vi "rs3 init all2.vi"(8 "error in":errorcluster, 10 "Select Device":i32, 11 "Select Sensor":i32) -> (0 "error out":errorcluster, 1 "Adv. enable?":i32, 2 "init results":T3, 3 "init error":string, 4 "All Devices":T2(array[cluster]), 5 "Sensor Array":T1(array[cluster]), 7 "Found RealSense":bool)   [LabVIEW 2019, in "libRealSense3.lvlib"]
doc: "Initialized the RealSense device. \nSelect the specific DEVICE and its specific SENSOR. \n\n\nINPUT:\nSelect Device The INDEX to the specific DEVICE handle\nSelect Sensor The INDEX to the specific SENSOR that is part of the selected DEVICE.\n \nOUTPUT:\ninit result Contains all the information about the selected device and its sensor. You will need to use the Dev Out HANDLE to communicate with the device. \n \nselected sensor array Contains the arrays of SENSORS attached to a specific DEVICE.\nall devices Contains array of all device that are attached to the PC."
uses:
  libRealSense3.lvlib
panel:
  # "RS3 Init All"
  # "(C) Intel Corp. 2017,  AGJ"
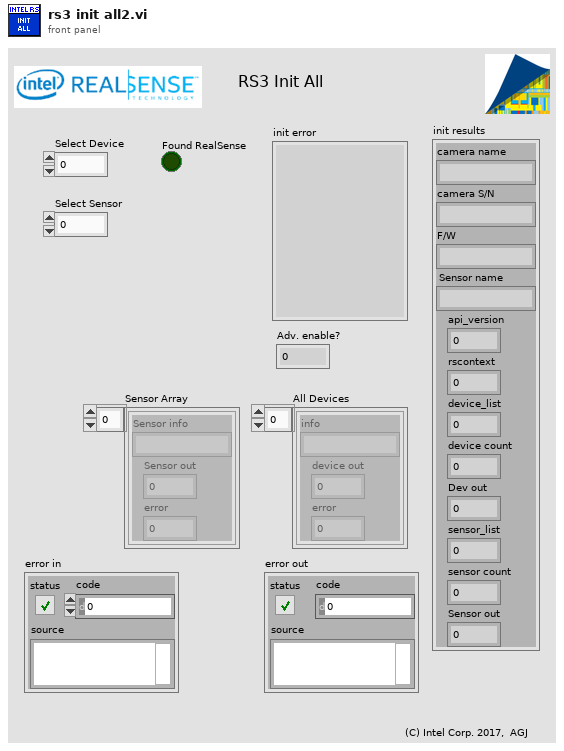
[diagram p1: front panel]
types:
  T1 = cluster{"Sensor info":string, "Sensor out":u64, "error":u64}[]
  T2 = cluster{"info":string, "device out":u64, "error":u64}[]
  T3 = cluster{"camera name":string, "camera S/N":string, "F/W":string, "Sensor name":string, "api_version":i32, "rscontext":u64, "device_list":u64, "device count":i32, "Dev out":u64, "sensor_list":u64, "sensor count":i32, "Sensor out":u64}
  T4 = cluster{"info":string, "device out":u64, "error":u64}
  T5 = cluster{"info":string, "info":string, "info":string, "Sensor info":string, "api_version":i32, "rscontext":u64, "device_list":u64, "device count":i32, "device out":u64, "sensor_list":u64, "sensor count":i32, "Sensor out":u64}
  T6 = cluster{"Sensor info":string, "Sensor out":u64, "error":u64}
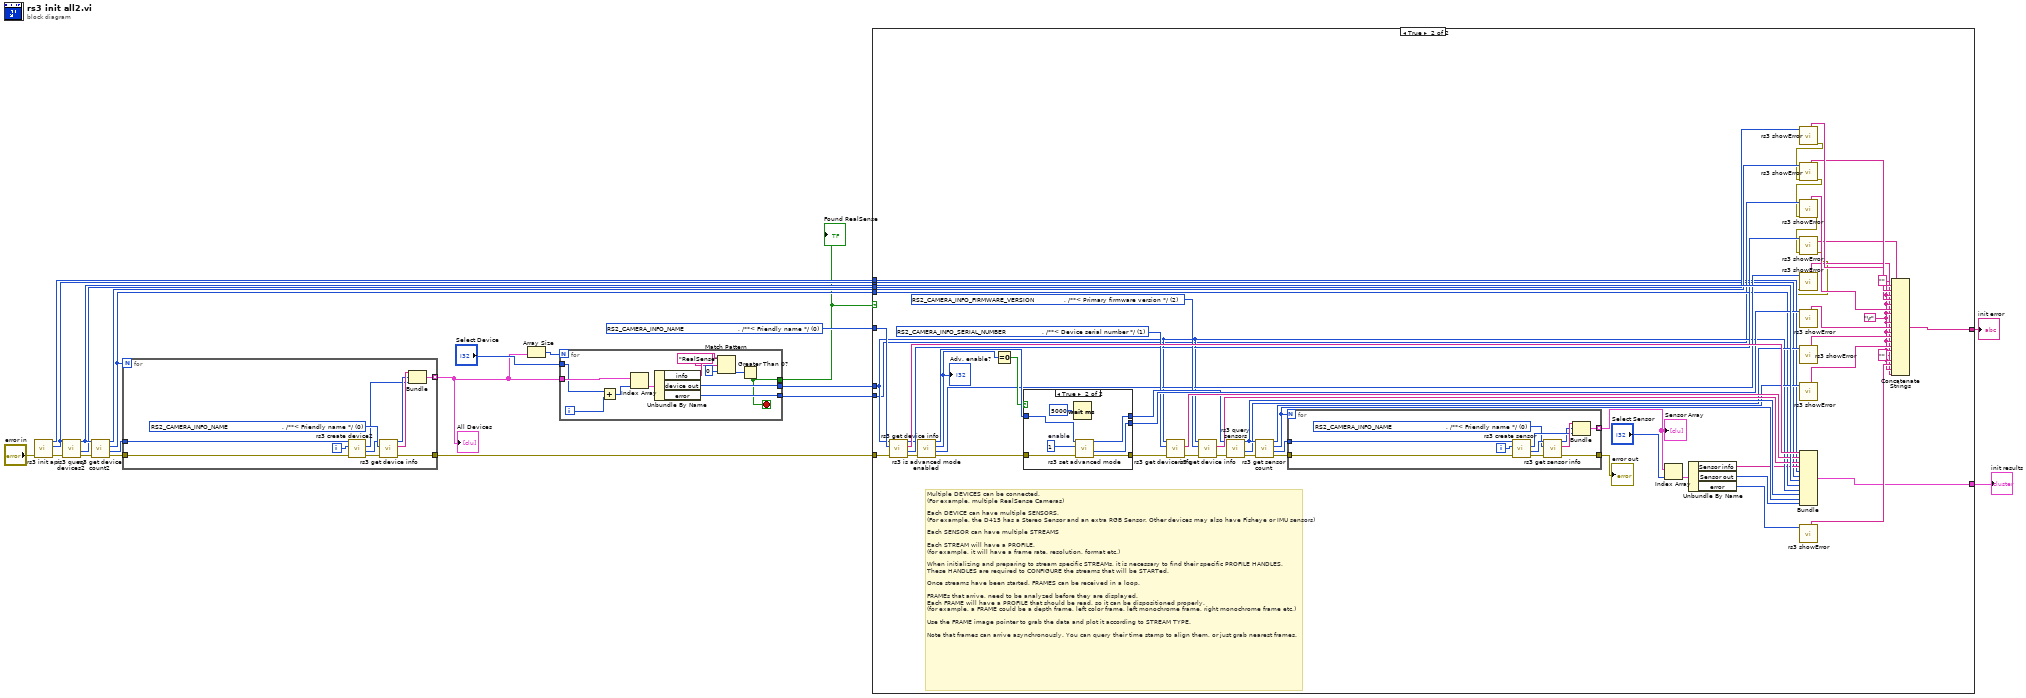
[diagram p0: block diagram]
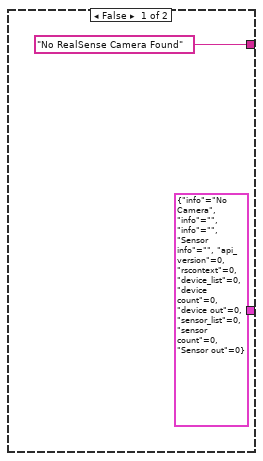
[diagram p2: hidden frame]
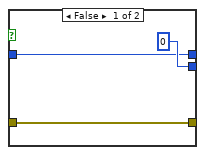
[diagram p3: hidden frame]
diagram:
  w20 = u16 0 items=["    RS2_CAMERA_INFO_NAME                           , /**< Friendly name */", "    RS2_CAMERA_INFO_SERIAL_NUMBER                  , /**< Device serial number */", "    RS2_CAMERA_INFO_FIRMWARE_VERSION               , /**< Primary firmware version */", "    RS2_CAMERA_INFO_PHYSICAL_PORT                       , /**< Unique identifier of the port the device is connected to (platform specific) */", "    RS2_CAMERA_INFO_DEBUG_OP_CODE                  , /**< If device supports firmware logging, this is the command to send to get logs from firmware */", "    RS2_CAMERA_INFO_ADVANCED_MODE                  , /**< True iff the device is in advanced mode */", "    RS2_CAMERA_INFO_PRODUCT_ID                     , /**< Product ID as reported in the USB descriptor */", "    RS2_CAMERA_INFO_CAMERA_LOCKED                  , /**< True iff EEPROM is locked */", "    RS2_CAMERA_INFO_COUNT                            /**< Number of enumeration values. Not a valid input: intended to be used in for-loops. */"] ("RS Camera info")
  n1 = call "rs3 init api.vi"("error in (no error)"="error in") -> ("error out"=w9:errorcluster, "rscontext"=w7:u64, "api_version"=w6:i32)  [unwired: 7 in, 1 out]
  n2 = call "rs3 query devices2.vi"("error in (no error)"=w9, "rscontext"=w7) -> ("error out"=w18:errorcluster, "error"=w17:u64, "device_list"=w21:u64)  [unwired: 7 in]
  n3 = call "rs3 get device count2.vi"("error in"=w18, "device_list"=w21) -> ("error out"=w12:errorcluster, "device_list_out"=w15:u64, "device count"=w16:i32, "error"=w19:u64)  [unwired: 6 in]
  n4 = for {
    N: w16 -> [_]
    tunnel: w15 -> [w32]
    tunnel: [w26] -> w1 mode=indexing
    tunnel: w12 -> [w25]
    tunnel: [w24] -> w11
    i -> [w31]
    w29 = u16 0 items=["    RS2_CAMERA_INFO_NAME                           , /**< Friendly name */", "    RS2_CAMERA_INFO_SERIAL_NUMBER                  , /**< Device serial number */", "    RS2_CAMERA_INFO_FIRMWARE_VERSION               , /**< Primary firmware version */", "    RS2_CAMERA_INFO_PHYSICAL_PORT                       , /**< Unique identifier of the port the device is connected to (platform specific) */", "    RS2_CAMERA_INFO_DEBUG_OP_CODE                  , /**< If device supports firmware logging, this is the command to send to get logs from firmware */", "    RS2_CAMERA_INFO_ADVANCED_MODE                  , /**< True iff the device is in advanced mode */", "    RS2_CAMERA_INFO_PRODUCT_ID                     , /**< Product ID as reported in the USB descriptor */", "    RS2_CAMERA_INFO_CAMERA_LOCKED                  , /**< True iff EEPROM is locked */", "    RS2_CAMERA_INFO_COUNT                            /**< Number of enumeration values. Not a valid input: intended to be used in for-loops. */"] ("RS Camera info")
    n5 = call "rs3 create device2.vi"("error in (no error)"=w25, "Device index"=w31, "device list in"=w32) -> ("error out"=w30:errorcluster, "Dev out"=w23:u64, "error"=w22:u64)  [unwired: 5 in, 1 out]
    n6 = call "rs3 get device info.vi"("error in (no error)"=w30, "RS Camera info"=w29, "device in"=w23) -> ("error out"=w24:errorcluster, "info"=w28:string, "device out"=w27:u64)  [unwired: 5 in, 1 out]
    n7 = Bundle("info"=w28, "device out"=w27, "error"=w22) -> (w26:T4)  [unwired: 1 in]
  }
  "All Devices" <- w1
  n8 = Array Size(array=w1) -> (size(s)=w2:i32)
  n9 = for {
    N: w2 -> [_]
    tunnel: w1 -> [w44]
    tunnel: "Select Device" -> [w35]
    tunnel: [w42] -> w13
    tunnel: [w41] -> w10
    tunnel: [w33] -> w5
    i -> [w36]
    stop <- w33 stop-if-true
    n10 = Add(x=w35, y=w36) -> (x+y=w37:i32)
    n11 = Index Array(array=w44, index=w37) -> (element=w43:T4)
    n12 = Unbundle By Name(w43) -> ("info"=w39:string, "device out"=w42:u64, "error"=w41:u64)
    n13 = Match Pattern(string=w39, regular expression="RealSense" ("string"), offset (0)=0) -> (offset past match=w34:i32)  [unwired: 3 out]
    n14 = Greater Than 0?(x=w34) -> (x > 0?=w33:bool)
  }
  "Found RealSense" <- w5
  n15 = case shown="True" w5 {
    tunnel: w21 -> [_ w104]
    tunnel: w20 -> [_ w91]
    tunnel: w19 -> [_ w89]
    tunnel: w17 -> [_ w88]
    tunnel: w16 -> [_ w70]
    tunnel: w13 -> [_ w69]
    tunnel: w11 -> [_ w68]
    tunnel: w10 -> [_ w67]
    tunnel: w7 -> [_ w56]
    tunnel: w6 -> [_ w55]
    tunnel: ["No RealSense Camera Found" w54] -> w4
    tunnel: [T5 {"info"="No Camera", "info"="", "info"="", "Sensor info"="", "api_version"=0, "rscontext"=0, "device_list"=0, "device count"=0, "device out"=0, "sensor_list"=0, "sensor count"=0, "Sensor out"=0} w53] -> w3
    frame False {
    }
    frame True {
      w72 = "\r"
      w98 = u16 2 items=["    RS2_CAMERA_INFO_NAME                           , /**< Friendly name */", "    RS2_CAMERA_INFO_SERIAL_NUMBER                  , /**< Device serial number */", "    RS2_CAMERA_INFO_FIRMWARE_VERSION               , /**< Primary firmware version */", "    RS2_CAMERA_INFO_PHYSICAL_PORT                       , /**< Unique identifier of the port the device is connected to (platform specific) */", "    RS2_CAMERA_INFO_DEBUG_OP_CODE                  , /**< If device supports firmware logging, this is the command to send to get logs from firmware */", "    RS2_CAMERA_INFO_ADVANCED_MODE                  , /**< True iff the device is in advanced mode */", "    RS2_CAMERA_INFO_PRODUCT_ID                     , /**< Product ID as reported in the USB descriptor */", "    RS2_CAMERA_INFO_CAMERA_LOCKED                  , /**< True iff EEPROM is locked */", "    RS2_CAMERA_INFO_COUNT                            /**< Number of enumeration values. Not a valid input: intended to be used in for-loops. */"] ("RS Camera info")
      w97 = u16 1 items=["    RS2_CAMERA_INFO_NAME                           , /**< Friendly name */", "    RS2_CAMERA_INFO_SERIAL_NUMBER                  , /**< Device serial number */", "    RS2_CAMERA_INFO_FIRMWARE_VERSION               , /**< Primary firmware version */", "    RS2_CAMERA_INFO_PHYSICAL_PORT                       , /**< Unique identifier of the port the device is connected to (platform specific) */", "    RS2_CAMERA_INFO_DEBUG_OP_CODE                  , /**< If device supports firmware logging, this is the command to send to get logs from firmware */", "    RS2_CAMERA_INFO_ADVANCED_MODE                  , /**< True iff the device is in advanced mode */", "    RS2_CAMERA_INFO_PRODUCT_ID                     , /**< Product ID as reported in the USB descriptor */", "    RS2_CAMERA_INFO_CAMERA_LOCKED                  , /**< True iff EEPROM is locked */", "    RS2_CAMERA_INFO_COUNT                            /**< Number of enumeration values. Not a valid input: intended to be used in for-loops. */"] ("RS Camera info")
      # "Multiple DEVICES can be connected. \n(For example, multiple RealSense Cameras)\n\nEach DEVICE can have multiple SENSORS. \n(For example, the D415 has a Stereo Sensor and an extra RGB Sensor. Other devices may also have Fisheye or IMU sensors) \n\nEach SENSOR can have multiple STREAMS\n\nEach STREAM will have a PROFILE. \n(for example, it will have a frame rate, resolution, format etc.)\n\nWhen initializing and preparing to stream specific STREAMs, it is necessary to find their specific PROFILE HANDLES.\nThese HANDLES are required to CONFIGURE the streams that will be STARTed. \n\nOnce streams have been started, FRAMES can be received in a loop. \n \nFRAMEs that arrive, need to be analyzed before they are displayed. \nEach FRAME will have a PROFILE that should be read, so it can be dispositioned properly.\n(for example, a FRAME could be a depth frame, left color frame, left monochrome frame, right monochrome frame etc.)\n\nUse the FRAME image pointer to grab the data and plot it according to STREAM TYPE.\n\nNote that frames can arrive asynchronously. You can query their time stamp to align them, or just grab nearest frames."
      n16 = call "rs3 get device info.vi"("error in (no error)"=w68, "RS Camera info"=w91, "device in"=w69) -> ("error out"=w79:errorcluster, "error"=w90:u64, "info"=w105:string, "device out"=w77:u64)  [unwired: 5 in]
      n17 = call "rs3 is advanced mode enabled.vi"("error in (no error)"=w79, "device in"=w77) -> ("error out"=w78:errorcluster, "error"=w73:u64, "enable?"=w75:i32, "device out"=w76:u64)  [unwired: 6 in]
      "Adv. enable?" <- w75
      n18 = Equal To 0?(x=w75) -> (x = 0?=w74:bool)
      n19 = case shown="True" w74 {
        tunnel: [u64 0 ("error") w127] -> w101
        tunnel: [w118 w125] -> w100
        tunnel: w76 -> [w118 w124]
        tunnel: [w120 w123] -> w99
        tunnel: w78 -> [w120 w122]
        frame False {
        }
        frame True {
          w126 = 1  # enable
          n20 = Wait (ms)(milliseconds to wait=u32 5000) -> ()  [unwired: 1 out]
          n21 = call "rs3 set advanced mode.vi"("error in (no error)"=w122, "enable"=w126, "device in"=w124) -> ("error out"=w123:errorcluster, "error"=w127:u64, "device out"=w125:u64)  [unwired: 6 in]
        }
      }
      n22 = call "rs3 get device info.vi"("error in (no error)"=w99, "RS Camera info"=w97, "device in"=w69) -> ("error out"=w95:errorcluster, "info"=w102:string)  [unwired: 5 in, 2 out]
      n23 = call "rs3 get device info.vi"("error in (no error)"=w95, "RS Camera info"=w98, "device in"=w69) -> ("error out"=w96:errorcluster, "info"=w103:string)  [unwired: 5 in, 2 out]
      n24 = call "rs3 query sensors.vi"("error in (no error)"=w96, "device in"=w100) -> ("error out"=w93:errorcluster, "error"=w92:u64, "sensor_list"=w106:u64)  [unwired: 7 in]
      n25 = call "rs3 get sensor count.vi"("error in"=w93, "sensor_list"=w106) -> ("error out"=w65:errorcluster, "sensor_list_out"=w64:u64, "sensor count"=w66:i32, "error"=w94:u64)  [unwired: 6 in]
      n26 = for {
        N: w66 -> [_]
        tunnel: w65 -> [w117]
        tunnel: w64 -> [w114]
        tunnel: [w108] -> w63 mode=indexing
        tunnel: [w107] -> w58
        i -> [w115]
        w110 = u16 0 items=["    RS2_CAMERA_INFO_NAME                           , /**< Friendly name */", "    RS2_CAMERA_INFO_SERIAL_NUMBER                  , /**< Device serial number */", "    RS2_CAMERA_INFO_FIRMWARE_VERSION               , /**< Primary firmware version */", "    RS2_CAMERA_INFO_PHYSICAL_PORT                       , /**< Unique identifier of the port the device is connected to (platform specific) */", "    RS2_CAMERA_INFO_DEBUG_OP_CODE                  , /**< If device supports firmware logging, this is the command to send to get logs from firmware */", "    RS2_CAMERA_INFO_ADVANCED_MODE                  , /**< True iff the device is in advanced mode */", "    RS2_CAMERA_INFO_PRODUCT_ID                     , /**< Product ID as reported in the USB descriptor */", "    RS2_CAMERA_INFO_CAMERA_LOCKED                  , /**< True iff EEPROM is locked */", "    RS2_CAMERA_INFO_COUNT                            /**< Number of enumeration values. Not a valid input: intended to be used in for-loops. */"] ("RS Sensor info")
        n27 = call "rs3 create sensor.vi"("error in (no error)"=w117, "Sensor index"=w115, "Sensor list"=w114) -> ("error out"=w116:errorcluster, "Sensor out"=w112:u64, "error"=w111:u64)  [unwired: 5 in, 1 out]
        n28 = call "rs3 get sensor info.vi"("error in (no error)"=w116, "RS Camera info"=w110, "Sensor in"=w112) -> ("error out"=w107:errorcluster, "Sensor info"=w113:string, "Sensor out"=w109:u64)  [unwired: 5 in, 1 out]
        n29 = Bundle("Sensor info"=w113, "Sensor out"=w109, "error"=w111) -> (w108:T6)  [unwired: 1 in]
      }
      "error out" <- w58
      "Sensor Array" <- w63
      n30 = Index Array(array=w63, index="Select Sensor") -> (element=w61:T6)
      n31 = Unbundle By Name(w61) -> ("Sensor info"=w57:string, "Sensor out"=w60:u64, "error"=w59:u64)
      n32 = Bundle("info"=w105, "info"=w102, "info"=w103, "Sensor info"=w57, "api_version"=w55, "rscontext"=w56, "device_list"=w104, "device count"=w70, "device out"=w69, "sensor_list"=w106, "sensor count"=w66, "Sensor out"=w60) -> (w53:T5)  [unwired: 1 in]
      n33 = call "rs3 showError.vi"("error"=w88) -> ("error out"=w52:errorcluster, "Error summary"=w87:string)  [unwired: 6 in, 3 out]
      n34 = call "rs3 showError.vi"("error in (no error)"=w52, "error"=w89) -> ("error out"=w51:errorcluster, "Error summary"=w86:string)  [unwired: 5 in, 3 out]
      n35 = call "rs3 showError.vi"("error in (no error)"=w51, "error"=w67) -> ("error out"=w50:errorcluster, "Error summary"=w85:string)  [unwired: 5 in, 3 out]
      n36 = call "rs3 showError.vi"("error in (no error)"=w50, "error"=w90) -> ("error out"=w49:errorcluster, "Error summary"=w84:string)  [unwired: 5 in, 3 out]
      n37 = call "rs3 showError.vi"("error in (no error)"=w49, "error"=w73) -> ("Error summary"=w71:string)  [unwired: 5 in, 4 out]
      n38 = call "rs3 showError.vi"("error"=w101) -> ("Error summary"=w83:string)  [unwired: 6 in, 4 out]
      n39 = call "rs3 showError.vi"("error"=w92) -> ("Error summary"=w82:string)  [unwired: 6 in, 4 out]
      n40 = call "rs3 showError.vi"("error"=w94) -> ("Error summary"=w81:string)  [unwired: 6 in, 4 out]
      n41 = call "rs3 showError.vi"("error"=w59) -> ("Error summary"=w80:string)  [unwired: 6 in, 4 out]
      n42 = Concatenate Strings("" ("string"), w72, w87, w72, w86, w72, w85, w72, w84, w72, w83, w72, w82, w72, w81, w72, "" ("string"), w72, w80, w72, w71) -> (w54:string)
    }
  }
  "init error" <- w4
  "init results" <- w3
